vi "Raman Acquisition.vi"() -> ()   [LabVIEW 2009]
uses:
  <vilib>/Utility/error.llb/DialogType.ctl
  Raman.ctl
  <vilib>/DAQmx/configure/trigger.llb/DAQmx Start Trigger (Digital Edge).vi
  <vilib>/DAQmx/configure/timing.llb/DAQmx Timing (Sample Clock).vi
  <vilib>/DAQmx/create/channels.llb/DAQmx Create Channel (AI-Voltage-Basic).vi
  <vilib>/DAQmx/read.llb/DAQmx Read.vi
  <vilib>/DAQmx/read.llb/DAQmx Read (Analog 2D DBL NChan NSamp).vi
  <vilib>/Utility/file.llb/Write To Spreadsheet File (DBL).vi
  <vilib>/Analysis/NI_AALBase.lvlib
  <instrlib>/Agilent ESG Series/Agilent ESG Series.lvlib
panel:
  out "Current Frequency":dbl[unit]
  in  "Lower Threshold (% of Min)":dbl=120.0
  in  "Upper Threshold (% of Max)":dbl=80.0
  out "data":dbl[][](array[numeric]) format="%0.6f"
  out "Raman Measure":cluster{dbl[], dbl[]}[](graph)
  in  "Raman Measurement File":path=path "C:/Users/atomes/Desktop/Labview Projects/Raman Measure/raman.txt"
  in  "Scan Frequency":bool
  in  "Resonance Frequency":dbl[unit]=100000000.0
  out "Increment Count":i32
  in  "Start Frequency":dbl[unit]=-5000000.0
  in  "Stop Frequency":dbl[unit]=5000000.0
  in  "Number of Intervals":u32
  out "Frequency Interval":dbl[unit]
  in  "VISA session":refnum<visa-resource-name>="GPIB0::19::INSTR"
  in  "Number of Measurements":u32=10
  out "Acquisition Count":i32
  in  "Samples per Channel":i32=2048
  in  "stop":bool
  out "Measurement":dbl[][](graph) caption="Pulse Monitor"
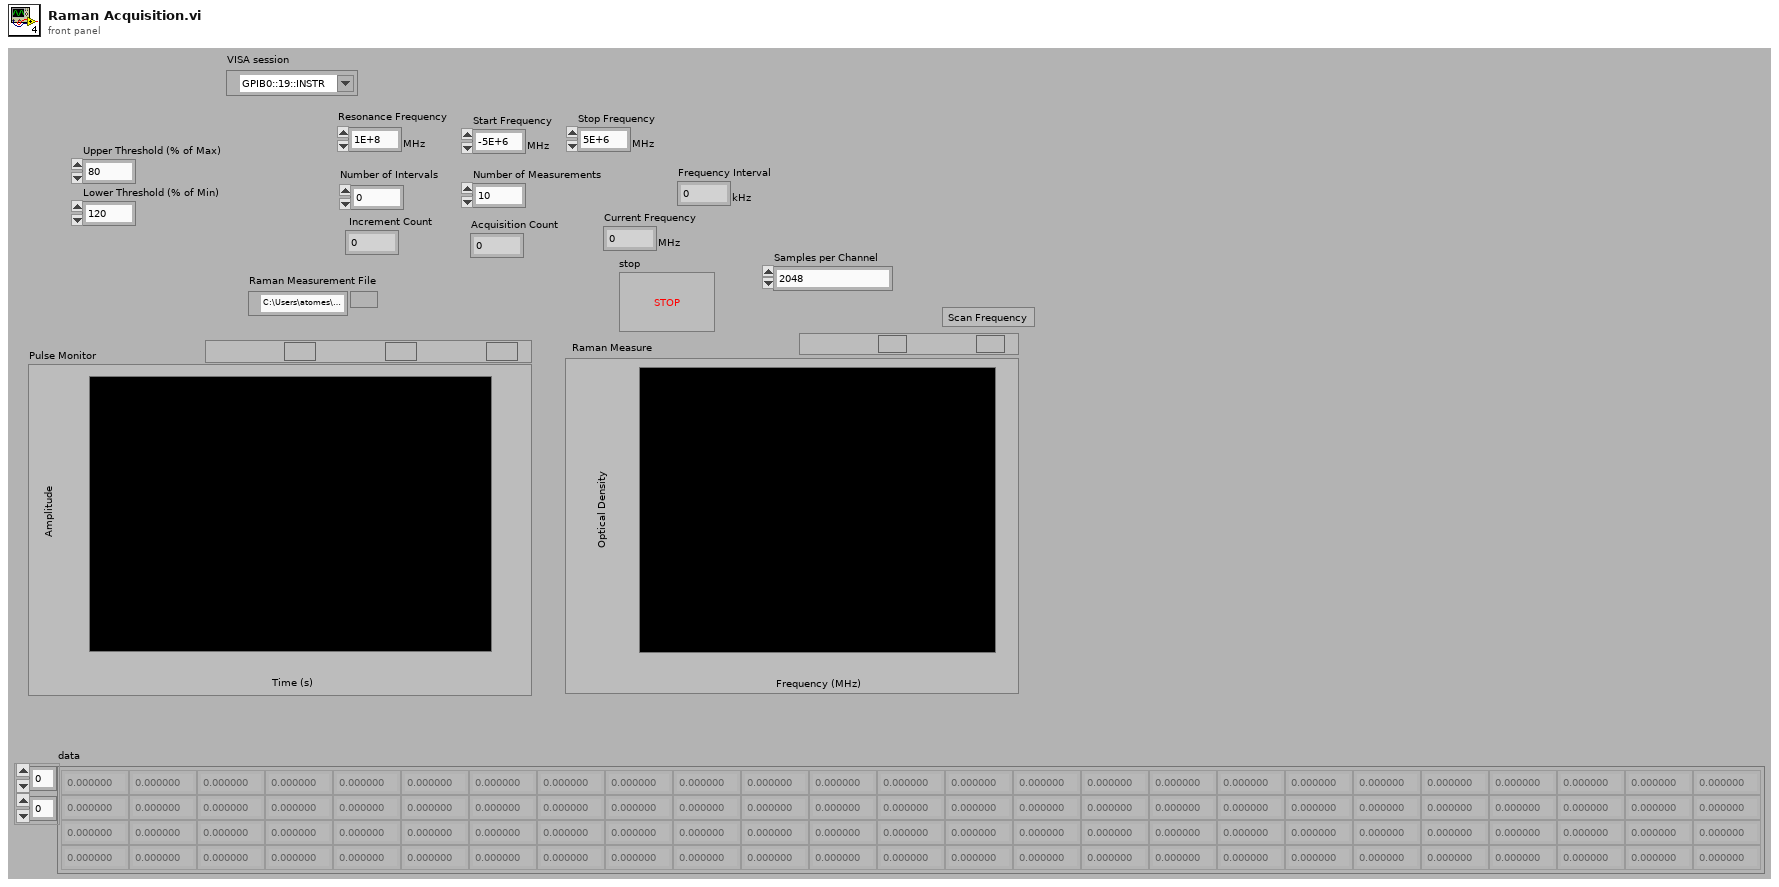
[diagram p1: front panel]
types:
  T1 = typedef "Raman.ctl" = enum16{"Initialize", "Monitor Pulses", "Scan Frequency", "Output Data", "Exit"}
  T2 = typedef "DialogType.ctl" = u16
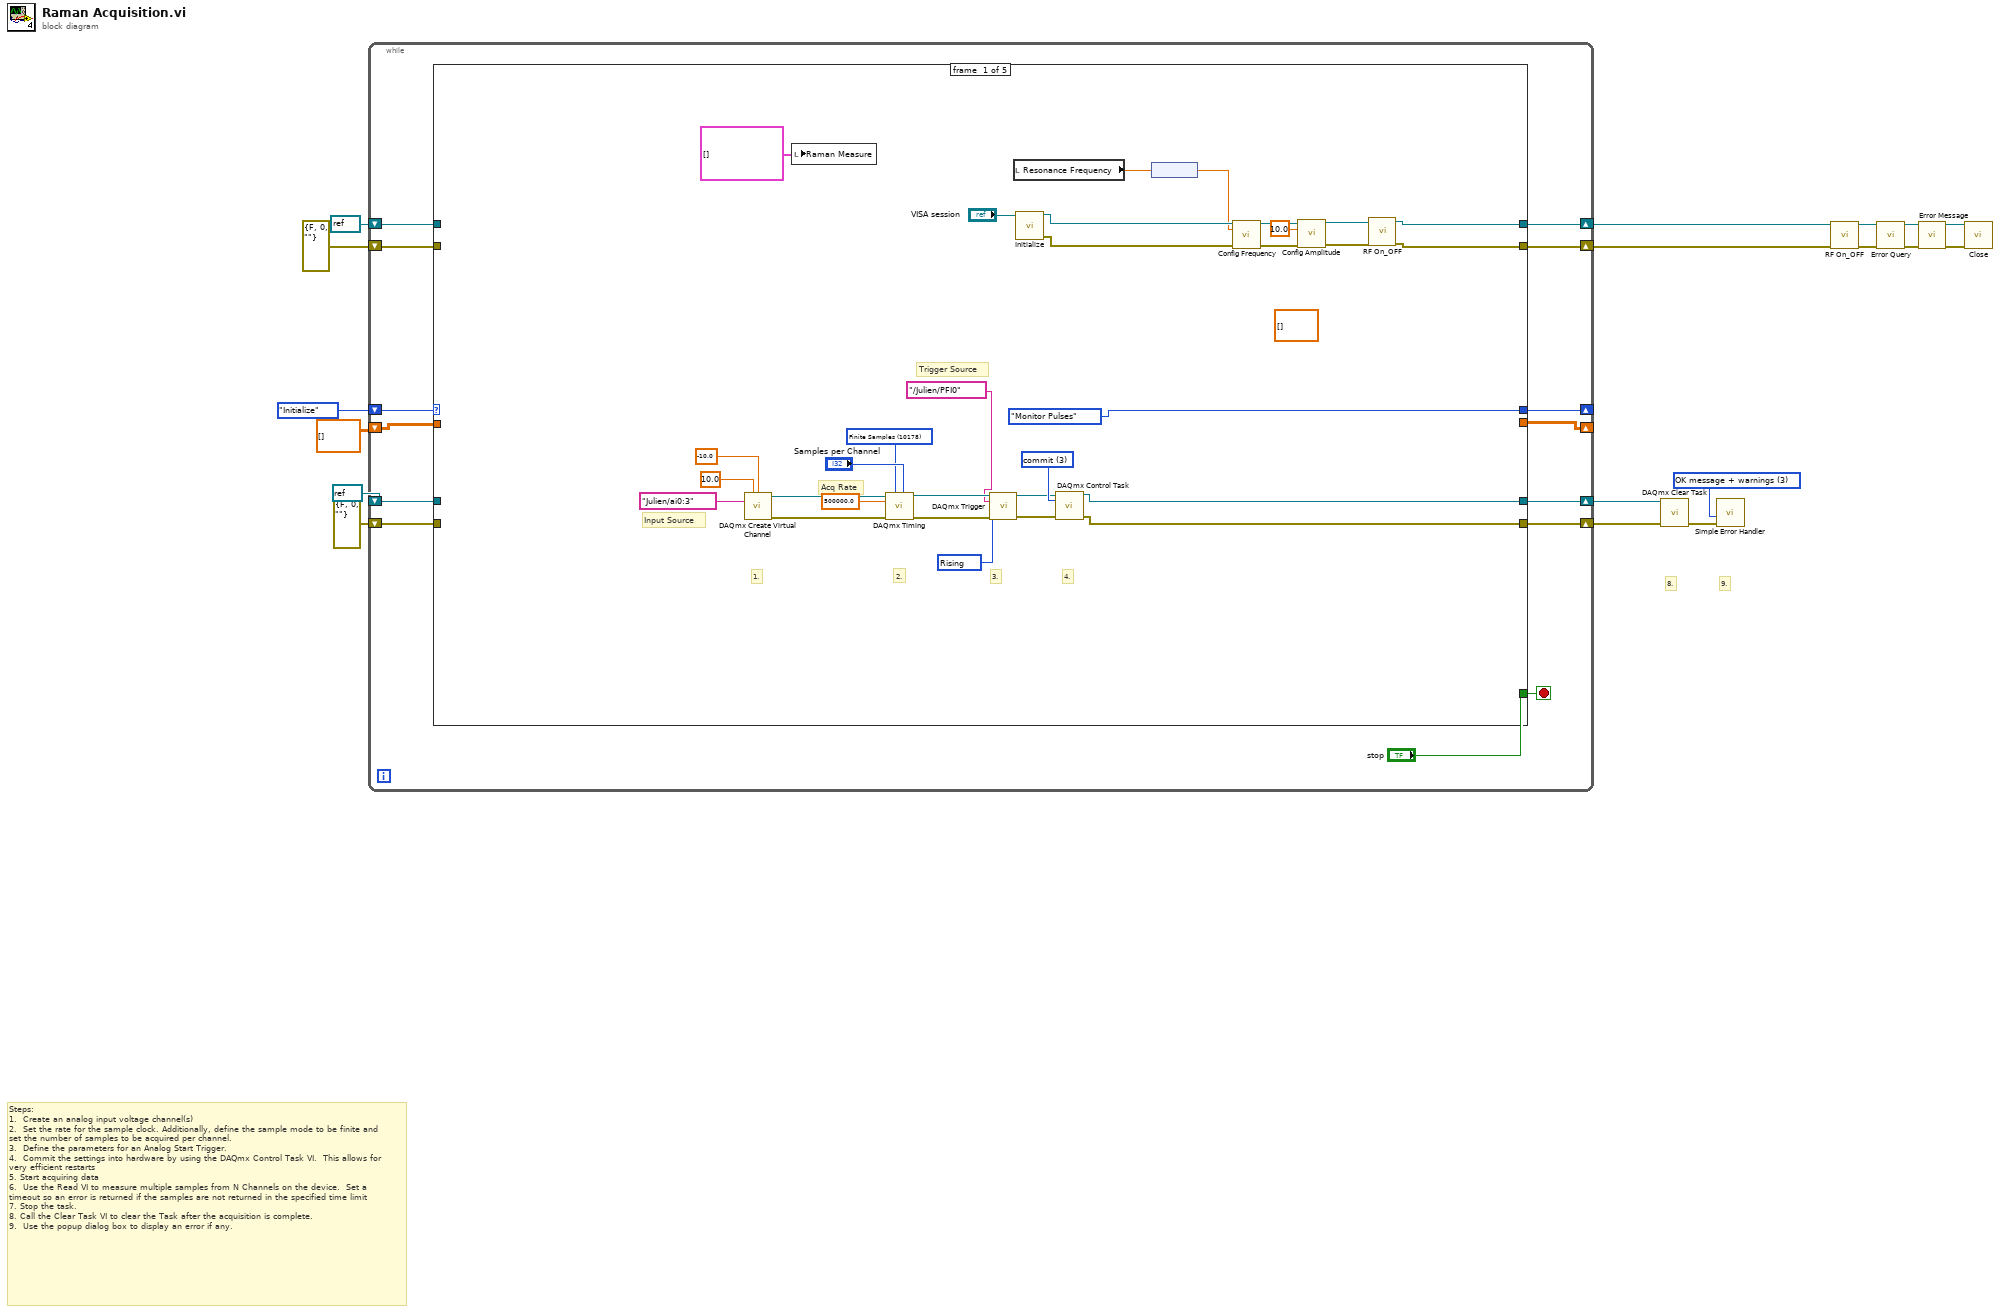
[diagram p0: block diagram]
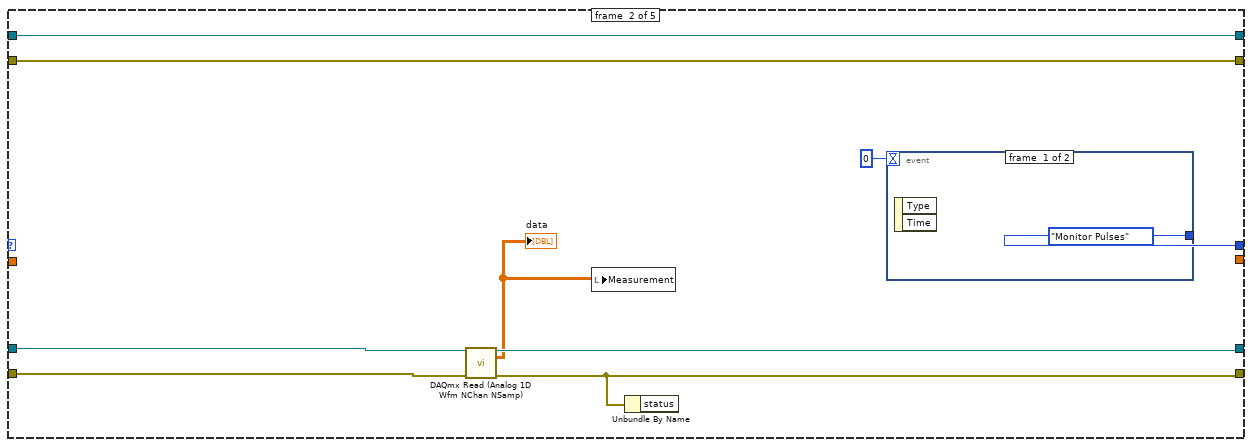
[diagram p2: hidden frame]
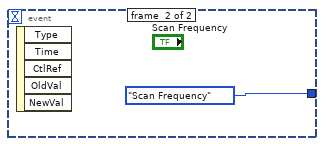
[diagram p3: hidden frame]
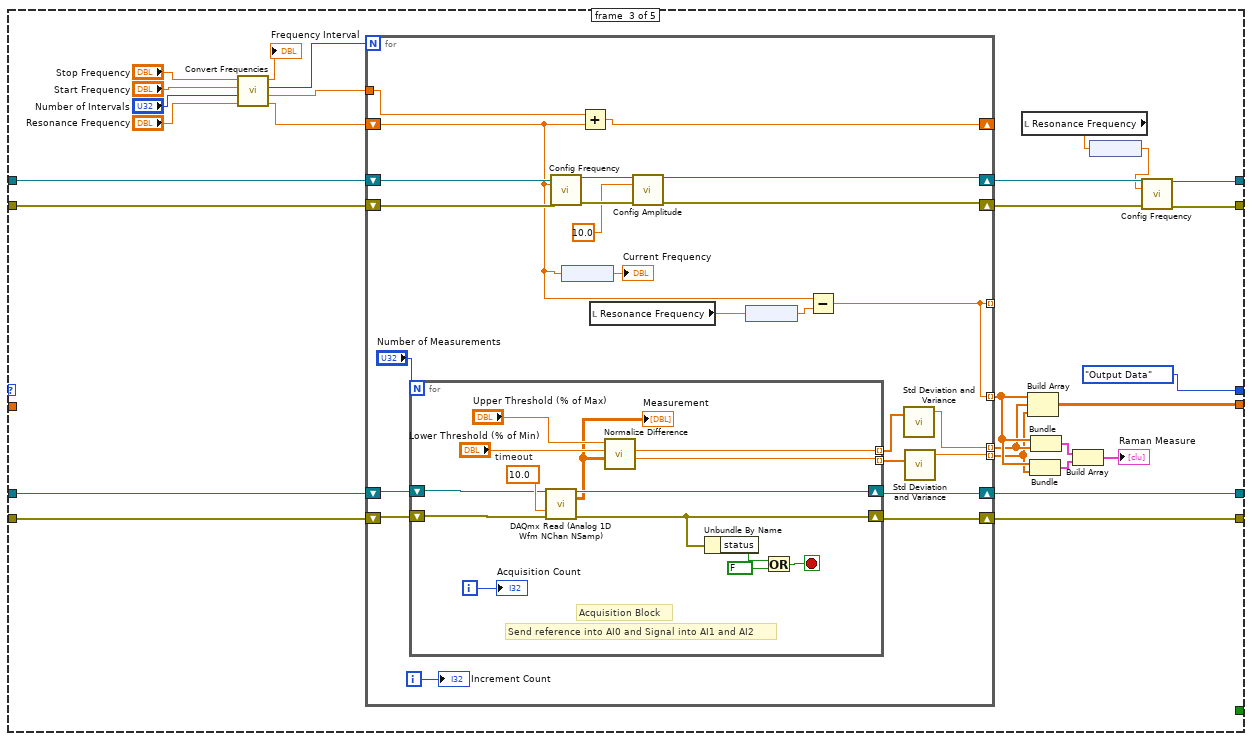
[diagram p4: hidden frame]
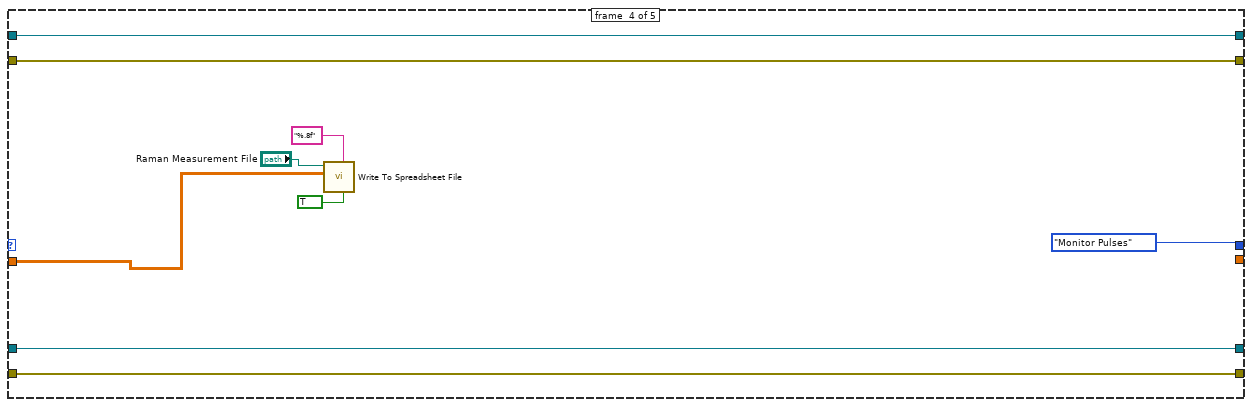
[diagram p5: hidden frame]
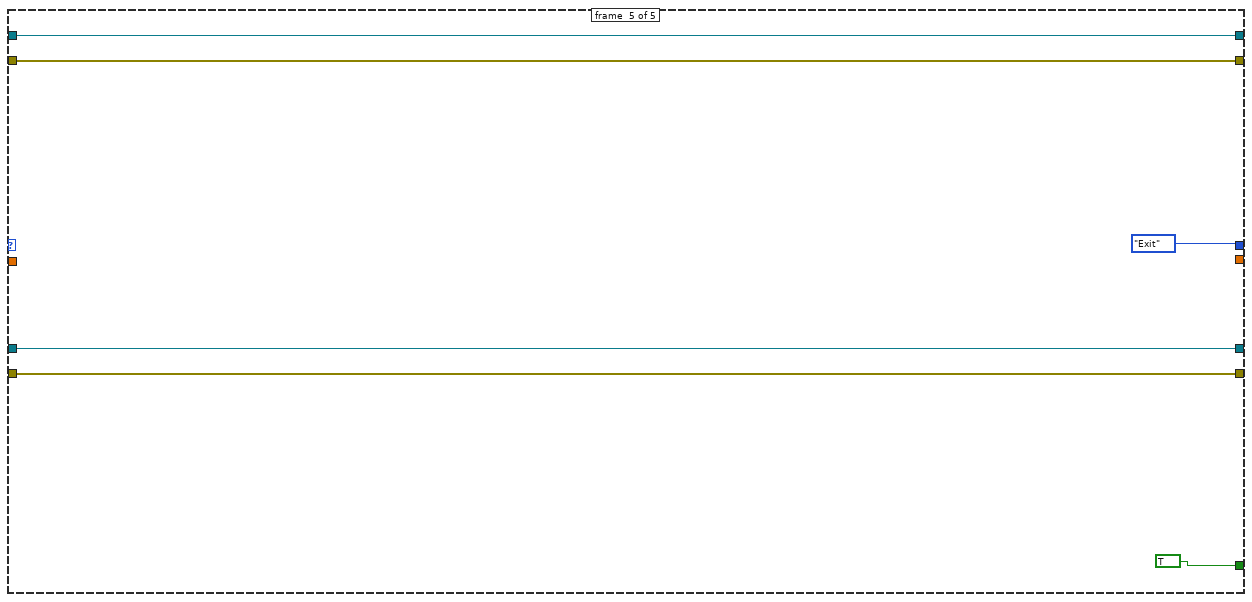
[diagram p6: hidden frame]
diagram:
  w16 = T2 3 items=["no dialog", "OK message", "continue or stop message", "OK message + warnings", "continue/stop + warnings"] ("type of dialog (OK msg:1)")
  # "9."
  # "8."
  # "Steps: \n1.  Create an analog input voltage channel(s)\n2.  Set the rate for the sample clock. Additionally, define the sample mode to be finite and set the number of samples to be acquired per channel.\n3.  Define the parameters for an Analog Start Trigger.\n4.  Commit the settings into hardware by using the DAQmx Control Task VI.  This allows for very efficient restarts\n5. Start acquiring data\n6.  Use the Read VI to measure multiple samples from N Channels on the device.  Set a timeout so an error is returned if the samples are not returned in the specified time limit\n7. Stop the task.\n8. Call the Clear Task VI to clear the Task after the acquisition is complete.\n9.  Use the popup dialog box to display an error if any."
  n1 = while {
    shift-right: [w26] -> _
    shift-left: Raman."Initialize" ("Raman State") -> [w27]
    shift-right: [w30] -> w17
    shift-left: refnum<k21> refnum ("task out") -> [w25]
    shift-right: [w31] -> w18
    shift-left: errorcluster {"status"=FALSE, "code"=0, "source"=""} ("error out") -> [w24]
    shift-right: [w19] -> _
    shift-left: dbl[][] [] -> [w23]
    shift-right: [w28] -> w1
    shift-left: refnum<visa-resource-name> refnum ("VISA Resource Name Out") -> [w22]
    shift-right: [w29] -> w14
    shift-left: errorcluster {"status"=FALSE, "code"=0, "source"=""} ("error out") -> [w21]
    stop <- "stop" stop-if-true
    n2 = case shown="\"Scan Frequency\"" w27 {
      tunnel: [w46 w64 w101 w142 w150] -> w31
      tunnel: [w47 w65 w100 w143 w151] -> w30
      tunnel: [w34 w69 w86 w140 w152] -> w29
      tunnel: [w33 w70 w87 w141 w153] -> w28
      tunnel: [Raman."Monitor Pulses" ("Raman State") w71 Raman."Output Data" ("Raman State") Raman."Monitor Pulses" ("Raman State") Raman."Exit" ("Raman State")] -> w26
      tunnel: w25 -> [_ w67 w93 w143 w151]
      tunnel: w24 -> [_ w66 w92 w142 w150]
      tunnel: w23 -> [_ _ _ w146 _]
      tunnel: w22 -> [_ w70 w90 w141 w153]
      tunnel: w21 -> [_ w69 w89 w140 w152]
      tunnel: [_ _ _ _ TRUE] -> _
      tunnel: [_ _ w74 _ _] -> w19
      frame #0 {
        (unwired) dbl[][] [] ("Frequency/Delta Pairs")
        w62 = 10280 items=["Rising"=10280, "Falling"=10171] ("edge")
        w53 = 3 items=["verify"=2, "reserve"=4, "commit"=3, "unreserve"=5, "abort"=6] ("action")
        w54 = 10178 items=["Finite Samples"=10178, "Continuous Samples"=10123] ("sample mode")
        # "Input Source"
        # "Acq Rate"
        # "Trigger Source"
        # "4."
        # "3."
        # "2."
        # "1."
        n3 = call-poly <vilib>:"DAQmx Create Virtual Channel.vi"("maximum value"=10.0 ("Maximum Value"), "minimum value"=-10.0 ("Minimum Value"), "physical channels"=tag "Julien/ai0:3" ("Physical Channel")) -> ("task out"=w56:refnum<k21>, "error out"=w59:errorcluster)  [unwired: 11 in]
        n4 = local write "Raman Measure"(cluster{dbl[], dbl[]}[] [] ("Raman Measure")) -> ()
        n5 = call-poly <vilib>:"DAQmx Timing.vi"("task/channels in"=w56, "sample mode"=w54, "samples per channel"="Samples per Channel", "rate"=500000.0 ("Rate"), "error in"=w59) -> ("task out"=w52:refnum<k21>, "error out"=w51:errorcluster)  [unwired: 9 in]
        n6 = call-poly <vilib>:"DAQmx Trigger.vi"("task/channels in"=w52, "source"=tag "/Julien/PFI0" ("Trigger source"), "edge"=w62, "error in"=w51) -> ("task out"=w50:refnum<k21>, "error out"=w49:errorcluster)  [unwired: 10 in]
        n7 = local read "Resonance Frequency"() -> (w41:dbl[unit])
        n8 = call <instrlib>:"Initialize.vi"("VISA Resource Name"="VISA session") -> ("VISA Resource Name Out"=w43:refnum<visa-resource-name>, "error out"=w42:errorcluster)  [unwired: 4 in, 9 out]
        n9 = call <vilib>:"DAQmx Control Task.vi"("task/channels in"=w50, "action"=w53, "error in"=w49) -> ("task out"=w47:refnum<k21>, "error out"=w46:errorcluster)  [unwired: 11 in]
        n10 = node(w41) -> (w40:dbl)
        n11 = call <instrlib>:"Config Frequency.vi"("VISA Resource Name"=w43, "Frequency (1000.0)"=w40, "error in (no error)"=w42) -> ("VISA Resource Name Out"=w39:refnum<visa-resource-name>, "error out"=w38:errorcluster)  [unwired: 6 in, 5 out]
        n12 = call <instrlib>:"Config Amplitude.vi"("VISA Resource Name"=w39, "Amplitude (-135.00)"=10.0, "error in (no error)"=w38) -> ("VISA Resource Name Out"=w36:refnum<visa-resource-name>, "error out"=w35:errorcluster)  [unwired: 5 in, 6 out]
        n13 = call <instrlib>:"RF On_OFF.vi"("VISA Resource Name"=w36, "error in (no error)"=w35) -> ("VISA Resource Name Out"=w33:refnum<visa-resource-name>, "error out"=w34:errorcluster)  [unwired: 1 in, 11 out]
      }
      frame #1 {
        n14 = call-poly "DAQmx Read (Analog 1D Wfm NChan NSamp).vi"("task/channels in"=w67, "error in"=w66) -> ("task out"=w65:refnum<k21>, "data"=w63:dbl[][], "error out"=w64:errorcluster)  [unwired: 11 in]
        "data" <- w63
        n15 = local write "Measurement"(w63) -> ()
        n16 = Unbundle By Name(w64) -> ()  [unwired: 1 out]
        n17 = event shown="[1] \"Scan Frequency\": Value Change" {
          selector: _ -> [_ _]
          dyn-events: _ -> [_ _]
          timeout: 0 -> [_ _]
          tunnel: [Raman."Monitor Pulses" ("Raman State") Raman."Scan Frequency" ("Raman State")] -> w71
          event #0 {
            n18 = event-data() -> ()  [unwired: 1 in, 2 out]
          }
          event #1 {
            n19 = event-data() -> ()  [unwired: 1 in, 5 out]
          }
        }
      }
      frame #2 {
        n20 = call "Convert Frequencies.vi"("Resonance Frequency (MHz)"="Resonance Frequency", "Number of Intervals"="Number of Intervals", "Start Frequency (MHz)"="Start Frequency", "Stop Frequency (MHz)"="Stop Frequency") -> ("Start Frequency (Number)"=w95:dbl, "Frequency Increment (Number)"=w96:dbl, "Number of Intervals (Out)"=w97:u32, "Frequency Interval"=→"Frequency Interval":dbl[unit])
        n21 = for {
          N: w97 -> [_]
          shift-right: [w124] -> w100
          shift-left: w93 -> [w122]
          shift-right: [w125] -> w101
          shift-left: w92 -> [w123]
          tunnel: w96 -> [w119]
          shift-right: [w112] -> _
          shift-left: w95 -> [w103]
          shift-right: [w114] -> w88
          shift-left: w90 -> [w118]
          shift-right: [w113] -> w85
          shift-left: w89 -> [w117]
          tunnel: [w116] -> w76 mode=indexing
          tunnel: [w104] -> w77 mode=indexing
          tunnel: [w107] -> w75 mode=indexing
          tunnel: [w104] -> _ mode=indexing
          i -> [w115]
          n22 = for {
            N: "Number of Measurements" -> [_]
            shift-right: [w130] -> w124
            shift-left: w122 -> [w132]
            shift-right: [w129] -> w125
            shift-left: w123 -> [w131]
            tunnel: [w135] -> w120 mode=indexing
            tunnel: [w134] -> w108 mode=indexing
            i -> [w136]
            stop <- w137 stop-if-true
            w139 = 10.0  # timeout
            # "Acquisition Block"
            # "Send reference into AI0 and Signal into AI1 and AI2"
            n23 = call-poly "DAQmx Read (Analog 1D Wfm NChan NSamp).vi"("task/channels in"=w132, "timeout"=w139, "error in"=w131) -> ("task out"=w130:refnum<k21>, "data"=w126:dbl[][], "error out"=w129:errorcluster)  [unwired: 10 in]
            "Measurement" <- w126
            n24 = call "Normalize Difference.vi"("data"=w126, "Lower Threshold (% of Min)"="Lower Threshold (% of Min)", "Upper Threshold (% of Max)"="Upper Threshold (% of Max)") -> ("Normalized Difference (Reference - Signal 2)"=w134:dbl, "Normalized Difference  (Reference - Signal1)"=w135:dbl)  [unwired: 6 in, 1 out]
            n25 = Unbundle By Name(w129) -> ("status"=w138:bool)
            n26 = Or(x=w138, y=FALSE) -> (x .or. y?=w137:bool)
            "Acquisition Count" <- w136
          }
          n27 = call <instrlib>:"Config Frequency.vi"("VISA Resource Name"=w118, "Frequency (1000.0)"=w103, "error in (no error)"=w117) -> ("VISA Resource Name Out"=w110:refnum<visa-resource-name>, "error out"=w111:errorcluster)  [unwired: 6 in, 5 out]
          n28 = node(w103) -> (→"Current Frequency":dbl[unit])
          n29 = Add(x=w119, y=w103) -> (x+y=w112:dbl)
          n30 = local read "Resonance Frequency"() -> (w106:dbl[unit])
          n31 = call <instrlib>:"Config Amplitude.vi"("VISA Resource Name"=w110, "Amplitude (-135.00)"=10.0, "error in (no error)"=w111) -> ("VISA Resource Name Out"=w114:refnum<visa-resource-name>, "error out"=w113:errorcluster)  [unwired: 5 in, 6 out]
          n32 = node(w106) -> (w105:dbl)
          n33 = Subtract(x=w103, y=w105) -> (x-y=w104:dbl)
          n34 = call <vilib>:"Std Deviation and Variance.vi"("X"=w120) -> ("mean"=w116:dbl)  [unwired: 1 in, 2 out]
          n35 = call <vilib>:"Std Deviation and Variance.vi"("X"=w108) -> ("mean"=w107:dbl)  [unwired: 1 in, 2 out]
          "Increment Count" <- w115
        }
        n36 = local read "Resonance Frequency"() -> (w84:dbl[unit])
        n37 = Build Array(w77, w76, w75) -> (w74:dbl[][])
        n38 = Bundle(w77, w75) -> (w79:cluster{dbl[], dbl[]})  [unwired: 1 in]
        n39 = Bundle(w77, w76) -> (w80:cluster{dbl[], dbl[]})  [unwired: 1 in]
        n40 = Build Array(w80, w79) -> (→"Raman Measure":cluster{dbl[], dbl[]}[])
        n41 = node(w84) -> (w83:dbl)
        n42 = call <instrlib>:"Config Frequency.vi"("VISA Resource Name"=w88, "Frequency (1000.0)"=w83, "error in (no error)"=w85) -> ("VISA Resource Name Out"=w87:refnum<visa-resource-name>, "error out"=w86:errorcluster)  [unwired: 6 in, 5 out]
      }
      frame #3 {
        n43 = call-poly <vilib>:"Write To Spreadsheet File.vi"("transpose? (no:F)"=TRUE, "format (%.3f)"="%.8f", "2D data"=w146, "file path (dialog if empty)"="Raman Measurement File") -> ()  [unwired: 4 in, 1 out]
      }
      frame #4 {
      }
    }
  }
  n44 = call <vilib>:"DAQmx Clear Task.vi"("task in"=w17, "error in"=w18) -> ("error out"=w15:errorcluster)  [unwired: 13 in]
  n45 = call <vilib>:"Simple Error Handler.vi"("type of dialog (OK msg:1)"=w16, "error in (no error)"=w15) -> ()  [unwired: 3 in, 5 out]
  n46 = call <instrlib>:"RF On_OFF.vi"("VISA Resource Name"=w1, "error in (no error)"=w14) -> ("VISA Resource Name Out"=w10:refnum<visa-resource-name>, "error out"=w11:errorcluster)  [unwired: 1 in, 11 out]
  n47 = call <instrlib>:"Error Query.vi"("VISA Resource Name"=w10, "error in (no error)"=w11) -> ("VISA Resource Name Out"=w9:refnum<visa-resource-name>, "error out"=w12:errorcluster)  [unwired: 12 out]
  n48 = call <instrlib>:"Error Message.vi"("VISA Resource Name"=w9, "error in (no error)"=w12) -> ("VISA Resource Name Out"=w8:refnum<visa-resource-name>, "error out"=w13:errorcluster)  [unwired: 1 in, 11 out]
  n49 = call <instrlib>:"Close.vi"("VISA Resource Name"=w8, "error in (no error)"=w13) -> ()  [unwired: 14 out]
